vi "Listen For Msg Attributes.vi"(10 "Address":refnum<data-value>) -> (0 "Error out":errorcluster, 2 "Msg Attributes":refnum<data-value>)   [LabVIEW 2020, in "jettl.lvlib" / "Queue Transport.lvlib"]
uses:
  Queue Transport.lvlib
  Relation.ctl
  jettl.lvlib
  Teller.ctl
  Msg Attributes.ctl
  Msg Input/Msg Input.lvclass
  Msg Output/Msg Output.lvclass
  Msg/Msg.lvclass
  Transport/Transport.lvclass
  Actor/Actor.lvclass
  Msgs.ctl
  Unified Layer.ctl
  Actor Attributes.ctl
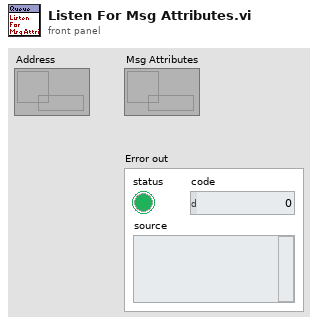
[diagram p1: front panel]
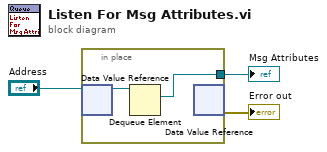
[diagram p0: block diagram]
diagram:
  n1 = in-place {
    in-place-border: [w4] -> w2
    n2 = in-place-dvr #1("Address") -> (w5:refnum<queue>)  [unwired: 1 out]
    n3 = Dequeue Element(queue=w5) -> (element=w4:refnum<data-value>)  [unwired: 2 in, 3 out]
    n4 = in-place-dvr #1() -> (→"Error out":errorcluster)  [unwired: 1 in, 1 out]
  }
  "Msg Attributes" <- w2
